vi "GlobalSettings.Create.vi"(8 "error in (no error)":errorcluster, 11 "Device Item Ref in":T1 format="%.0x") -> (0 "error out":errorcluster, 3 "Parent Ref out":T1 format="%.0x")   [LabVIEW 2019, in "Fuel Injector Analysis Addon System Explorer.lvlib"]
uses:
  Fuel Injector Analysis Addon System Explorer.lvlib
  <vilib>/NI VeriStand/Custom Device API/Custom Device Item Ref.ctl
  <vilib>/NI VeriStand/Custom Device API/Custom Device Channel.ctl
  <vilib>/NI VeriStand/Custom Device API/Custom Device Channel Type.ctl
  Addon Shared/SubVIs/Constants.vi
  <vilib>/NI VeriStand/Custom Device API/Custom Device API.lvlib
  Addon Shared/Fuel Injector Analysis Addon Shared.lvlib
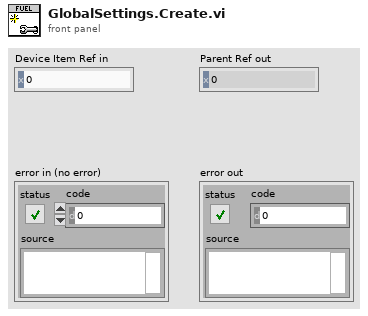
[diagram p1: front panel]
types:
  T1 = typedef "Custom Device API.lvlib/Custom Device Item Ref.ctl" = u64
  T2 = typedef "Custom Device API.lvlib/Custom Device Channel.ctl" = cluster{"Type":T3, "Units":string, "Default Value":dbl, "Faultable":bool, "Scalable":bool}
  T3 = typedef "Custom Device API.lvlib/Custom Device Channel Type.ctl" = enum16{"Input", "Output"}
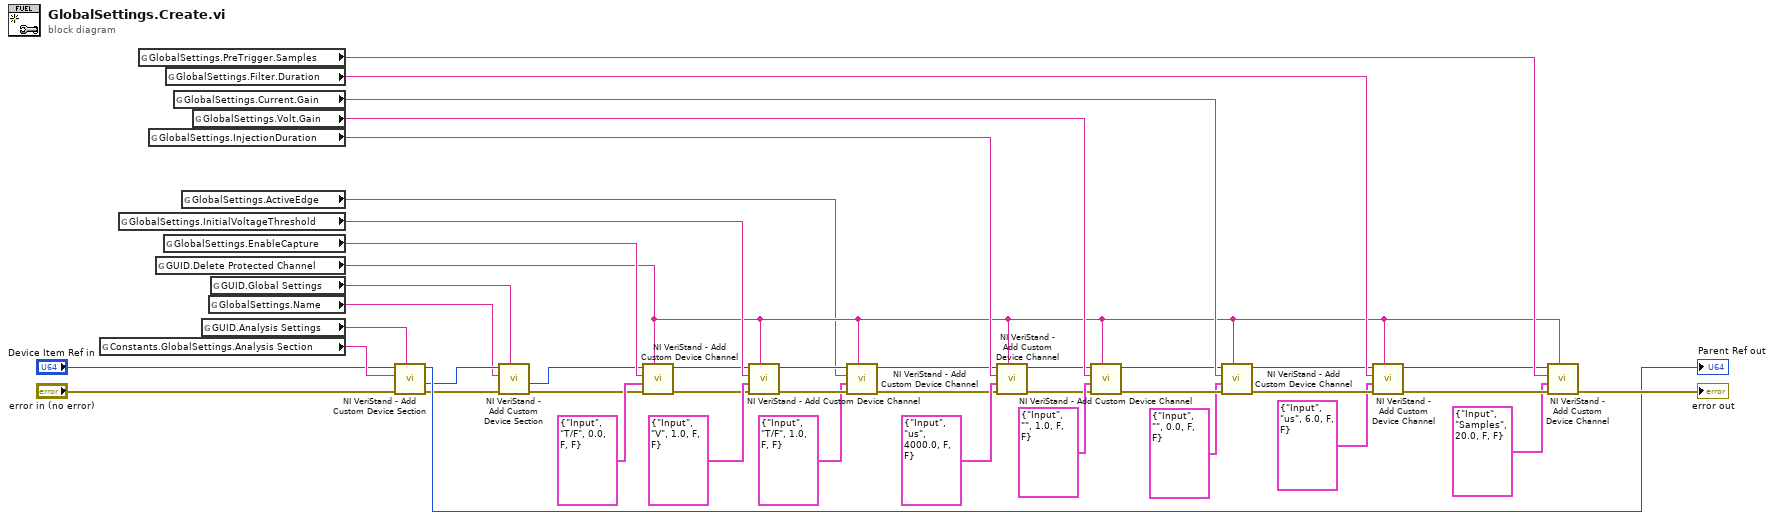
[diagram p0: block diagram]
diagram:
  n1 = global read "Constants.vi" "Constants.GlobalSettings.Analysis Section"() -> (w27:string)
  n2 = global read "Constants.vi" "GlobalSettings.InitialVoltageThreshold"() -> (w34:string)
  n3 = global read "Constants.vi" "GlobalSettings.PreTrigger.Samples"() -> (w43:string)
  n4 = global read "Constants.vi" "GlobalSettings.InjectionDuration"() -> (w21:string)
  n5 = global read "Constants.vi" "GUID.Delete Protected Channel"() -> (w2:string)
  n6 = global read "Constants.vi" "GlobalSettings.EnableCapture"() -> (w20:string)
  n7 = global read "Constants.vi" "GlobalSettings.Filter.Duration"() -> (w42:string)
  n8 = global read "Constants.vi" "GlobalSettings.Current.Gain"() -> (w23:string)
  n9 = global read "Constants.vi" "GlobalSettings.ActiveEdge"() -> (w1:string)
  n10 = global read "Constants.vi" "GlobalSettings.Volt.Gain"() -> (w22:string)
  n11 = global read "Constants.vi" "GUID.Analysis Settings"() -> (w28:string)
  n12 = global read "Constants.vi" "GlobalSettings.Name"() -> (w11:string)
  n13 = global read "Constants.vi" "GUID.Global Settings"() -> (w8:string)
  n14 = call <vilib>:"NI VeriStand - Add Custom Device Section.vi"("GUID (Default Section)"=w28, "error in (no error)"="error in (no error)", "Section Name"=w27, "Parent Ref in"="Device Item Ref in") -> ("error out"=w25:errorcluster, "Section Ptr"=w29:T1, "Parent Ref out"=→"Parent Ref out":T1)  [unwired: 4 in, 1 out]
  n15 = call <vilib>:"NI VeriStand - Add Custom Device Section.vi"("GUID (Default Section)"=w8, "error in (no error)"=w25, "Section Name"=w11, "Parent Ref in"=w29) -> ("error out"=w9:errorcluster, "Section Ptr"=w10:T1)  [unwired: 4 in, 2 out]
  n16 = call <vilib>:"NI VeriStand - Add Custom Device Channel.vi"("GUID (Default Channel)"=w2, "error in (no error)"=w9, "Channel"=T2 {"Type"=enum."Input", "Units"="T/F", "Default Value"=0.0, "Faultable"=FALSE, "Scalable"=FALSE}, "Channel Name"=w20, "Parent Ref in"=w10) -> ("error out"=w31:errorcluster, "Parent Ref out"=w32:T1)  [unwired: 3 in, 2 out]
  n17 = call <vilib>:"NI VeriStand - Add Custom Device Channel.vi"("GUID (Default Channel)"=w2, "error in (no error)"=w31, "Channel"=T2 {"Type"=enum."Input", "Units"="V", "Default Value"=1.0, "Faultable"=FALSE, "Scalable"=FALSE}, "Channel Name"=w34, "Parent Ref in"=w32) -> ("error out"=w7:errorcluster, "Parent Ref out"=w6:T1)  [unwired: 3 in, 2 out]
  n18 = call <vilib>:"NI VeriStand - Add Custom Device Channel.vi"("GUID (Default Channel)"=w2, "error in (no error)"=w7, "Channel"=T2 {"Type"=enum."Input", "Units"="T/F", "Default Value"=1.0, "Faultable"=FALSE, "Scalable"=FALSE}, "Channel Name"=w1, "Parent Ref in"=w6) -> ("error out"=w4:errorcluster, "Parent Ref out"=w5:T1)  [unwired: 3 in, 2 out]
  n19 = call <vilib>:"NI VeriStand - Add Custom Device Channel.vi"("GUID (Default Channel)"=w2, "error in (no error)"=w4, "Channel"=T2 {"Type"=enum."Input", "Units"="us", "Default Value"=4000.0, "Faultable"=FALSE, "Scalable"=FALSE}, "Channel Name"=w21, "Parent Ref in"=w5) -> ("error out"=w15:errorcluster, "Parent Ref out"=w14:T1)  [unwired: 3 in, 2 out]
  n20 = call <vilib>:"NI VeriStand - Add Custom Device Channel.vi"("GUID (Default Channel)"=w2, "error in (no error)"=w15, "Channel"=T2 {"Type"=enum."Input", "Units"="", "Default Value"=1.0, "Faultable"=FALSE, "Scalable"=FALSE}, "Channel Name"=w22, "Parent Ref in"=w14) -> ("error out"=w19:errorcluster, "Parent Ref out"=w18:T1)  [unwired: 3 in, 2 out]
  n21 = call <vilib>:"NI VeriStand - Add Custom Device Channel.vi"("GUID (Default Channel)"=w2, "error in (no error)"=w19, "Channel"=T2 {"Type"=enum."Input", "Units"="", "Default Value"=0.0, "Faultable"=FALSE, "Scalable"=FALSE}, "Channel Name"=w23, "Parent Ref in"=w18) -> ("error out"=w37:errorcluster, "Parent Ref out"=w38:T1)  [unwired: 3 in, 2 out]
  n22 = call <vilib>:"NI VeriStand - Add Custom Device Channel.vi"("GUID (Default Channel)"=w2, "error in (no error)"=w37, "Channel"=T2 {"Type"=enum."Input", "Units"="us", "Default Value"=6.0, "Faultable"=FALSE, "Scalable"=FALSE}, "Channel Name"=w42, "Parent Ref in"=w38) -> ("error out"=w39:errorcluster, "Parent Ref out"=w40:T1)  [unwired: 3 in, 2 out]
  n23 = call <vilib>:"NI VeriStand - Add Custom Device Channel.vi"("GUID (Default Channel)"=w2, "error in (no error)"=w39, "Channel"=T2 {"Type"=enum."Input", "Units"="Samples", "Default Value"=20.0, "Faultable"=FALSE, "Scalable"=FALSE}, "Channel Name"=w43, "Parent Ref in"=w40) -> ("error out"=→"error out":errorcluster)  [unwired: 3 in, 3 out]
